vi "Create And Register Generic Method Server Event.vi"(8 "error in":errorcluster, 11 "gRPCid server in":T1) -> (0 "error out":errorcluster, 2 "Generic Method Event":refnum<user-event>, 3 "gRPCid server out":T1)   [LabVIEW 2019, in "grpc-lvsupport.lvlib"]
uses:
  grpc-lvsupport.lvlib
  Shared/grpcId.ctl
  typeDefs/Generic Method Event Data.ctl
  <vilib>/Utility/error.llb/Error Cluster From Error Code.vi
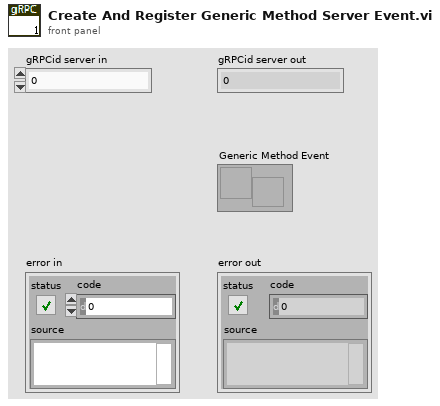
[diagram p1: front panel]
types:
  T1 = typedef "grpc-lvsupport.lvlib/grpcId.ctl" = u64
  T2 = typedef "grpc-lvsupport.lvlib/Generic Method Event Data.ctl" = cluster{"Method Name":string, "Method gRPCid":T1}
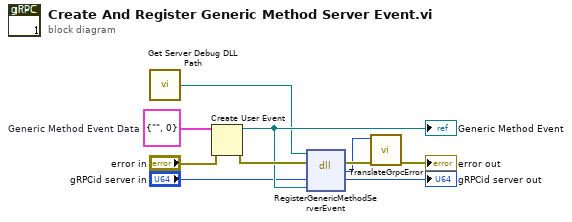
[diagram p0: block diagram]
diagram:
  w3 = T2 {"Method Name"="", "Method gRPCid"=0}  # Generic Method Event Data
  n1 = call "Get Server Debug DLL Path.vi"() -> ("Server dll path"=w4:path)
  n2 = Create User Event(user event datatype=w3, error in="error in") -> (user event=w7:refnum<user-event>, error out=w9:errorcluster)
  "Generic Method Event" <- w7
  n3 = dll-call lib="?" fn="RegisterGenericMethodServerEvent"(path in=w4, error in=w9, "serverId"="gRPCid server in", "genericMethodEvent"=w7) -> (error out=w8:errorcluster, "return type"=w1:i32, "serverId"=→"gRPCid server out":T1)  [unwired: 2 in, 1 out]
  n4 = call "TranslateGrpcError.vi"("error in"=w8, "Error Code"=w1) -> ("error out"=→"error out":errorcluster)  [unwired: 9 in]
